vi "ContourPlotIntoHistogram.vi"() -> ()   [LabVIEW 2017]
uses:
  <vilib>/Utility/file.llb/Read Delimited Spreadsheet (DBL).vi
  <vilib>/Utility/file.llb/Write Delimited Spreadsheet (I64).vi
  <vilib>/Utility/file.llb/Write Delimited Spreadsheet (DBL).vi
  <vilib>/Analysis/NI_AALPro.lvlib
panel:
  out "max value":dbl=0.9860422
  out "min value":dbl=0.1980103
  out "Progress %":dbl=99.37888198757764
  in  "intervals":i32=4000
  in  "book number":i32=375
  in  "file path (dialog if empty)":path=path "C:/Users/gyue/Box Sync/Guang Yue/data/Contour plot"
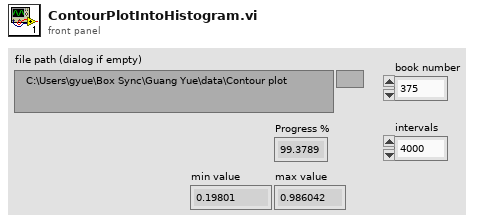
[diagram p1: front panel]
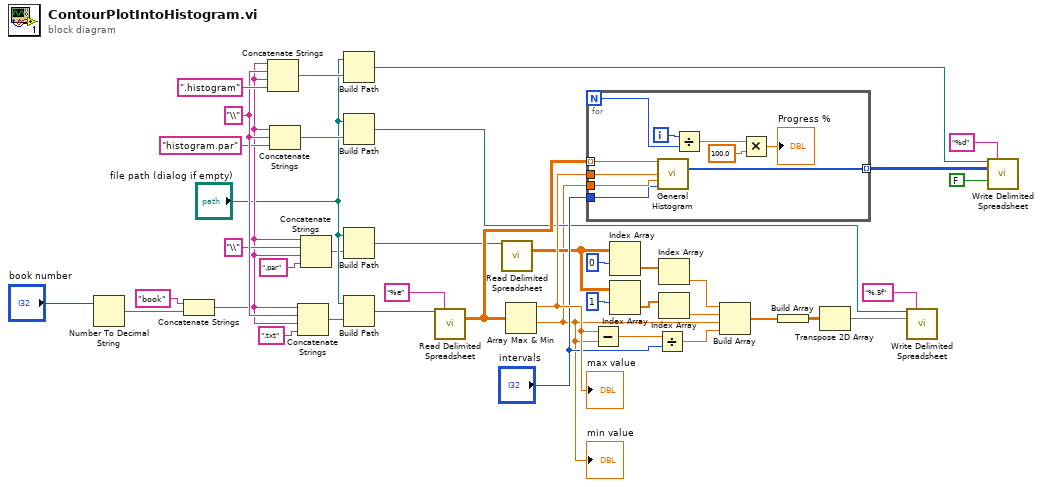
[diagram p0: block diagram]
diagram:
  w22 = "\\" ("string")
  n1 = Number To Decimal String(number="book number") -> (decimal integer string=w37:string)  [unwired: 1 in]
  n2 = Concatenate Strings("book" ("string"), w37) -> (w7:string)
  n3 = Concatenate Strings(w7, w22, w7, ".histogram" ("string")) -> (w26:string)
  n4 = Concatenate Strings(w7, w22, "histogram.par" ("string")) -> (w23:string)
  n5 = Concatenate Strings(w7, w22, w7, ".txt" ("string")) -> (w39:string)
  n6 = Concatenate Strings(w7, "\\" ("string"), w7, ".par" ("string")) -> (w5:string)
  n7 = Build Path(base path="file path (dialog if empty)", name or relative path=w26) -> (appended path=w25:path)
  n8 = Build Path(base path="file path (dialog if empty)", name or relative path=w23) -> (appended path=w17:path)
  n9 = Build Path(base path="file path (dialog if empty)", name or relative path=w5) -> (appended path=w15:path)
  n10 = Build Path(base path="file path (dialog if empty)", name or relative path=w39) -> (appended path=w40:path)
  n11 = call-poly <vilib>:"Read Delimited Spreadsheet.vi"("file path (dialog if empty)"=w40, "format (%.3f)"="%e") -> ("all rows"=w33:dbl[][])  [unwired: 8 in, 5 out]
  n12 = call-poly <vilib>:"Read Delimited Spreadsheet.vi"("file path (dialog if empty)"=w15) -> ("all rows"=w8:dbl[][])  [unwired: 9 in, 5 out]
  n13 = Array Max & Min(array=w33) -> (max value=w31:dbl, min value=w2:dbl)  [unwired: 2 out]
  "min value" <- w2
  "max value" <- w31
  n14 = for {
    N -> [w44]
    tunnel: w33 -> [w50] mode=indexing
    tunnel: w2 -> [w49]
    tunnel: w31 -> [w48]
    tunnel: "intervals" -> [w47]
    tunnel: [w46] -> w29 mode=indexing
    i -> [w45]
    n15 = call <vilib>:"General Histogram.vi"("X"=w50, "max"=w48, "min"=w49, "# bins"=w47) -> ("Histogram"=w46:i32[])  [unwired: 7 in, 4 out]
    n16 = Divide(x=w45, y=w44) -> (x/y=w43:dbl)
    n17 = Multiply(x=w43, y=100.0) -> (x*y=→"Progress %":dbl)
  }
  n18 = Subtract(x=w31, y=w2) -> (x-y=w32:dbl)
  n19 = Index Array(array=w8, index (row)=0) -> (element=w12:dbl[])  [unwired: 1 in]
  n20 = Index Array(array=w8, index (row)=1) -> (element=w11:dbl[])  [unwired: 1 in]
  n21 = Divide(x=w32, y="intervals") -> (x/y=w1:dbl)
  n22 = Index Array(array=w12) -> (element=w4:dbl)  [unwired: 1 in]
  n23 = Index Array(array=w11) -> (element=w3:dbl)  [unwired: 1 in]
  n24 = Build Array(w4, w3, w2, w1) -> (w20:dbl[])
  n25 = Build Array(w20) -> (w19:dbl[][])
  n26 = Transpose 2D Array(2D array=w19) -> (transposed array=w18:dbl[][])
  n27 = call-poly <vilib>:"Write Delimited Spreadsheet.vi"("file path (dialog if empty)"=w17, "format (%.3f)"="%.5f", "2D data"=w18) -> ()  [unwired: 11 in, 2 out]
  n28 = call-poly <vilib>:"Write Delimited Spreadsheet.vi"("file path (dialog if empty)"=w25, "format (%d)"="%d", "2D data"=w29, "append to file? (new file:F)"=FALSE) -> ()  [unwired: 10 in, 2 out]
